vi "mul_add_24_dc_ht_reg.vi"(4 "cep":bool, 8 "add":fxp<+/-,24,16> format="%#_10g", 10 "Signal":fxp<+/-,24,16>=32.0, 11 "coeff":fxp<+/-,18,2>=0.5) -> (1 "out":fxp<+/-,24,16>)   [LabVIEW 2018]
uses:
  <vilib>/rvi/FXPMathLib/basic elements/DSP48E/simVIs/niFpgaDsp48eSimulationState.ctl
  <vilib>/rvi/FXPMathLib/basic elements/DSP48E/subVIs/niFpgaDsp48eType.ctl
  <vilib>/rvi/FXPMathLib/basic elements/DSP48E/subVIs/niFpgaDsp48eAlumodeOpmodeCarryinselState.ctl
  <vilib>/rvi/FXPMathLib/basic elements/DSP48E/subVIs/niFpgaDsp48eUseMultiplierState.ctl
  <vilib>/rvi/FXPMathLib/basic elements/DSP48E/subVIs/niFpgaDsp48eLogicUnitModeState.ctl
  <vilib>/rvi/FXPMathLib/basic elements/DSP48E/subVIs/niFpgaDsp48eSelectPatternState.ctl
  <vilib>/rvi/FXPMathLib/basic elements/DSP48E/subVIs/niFpgaDsp48eSelectMaskState.ctl
  <vilib>/rvi/FXPMathLib/basic elements/DSP48E/subVIs/niFpgaDsp48eAutoresetState.ctl
  <vilib>/rvi/FXPMathLib/basic elements/DSP48E/simVIs/niFpgaDsp48eResets.ctl
  <vilib>/rvi/FXPMathLib/basic elements/DSP48E/simVIs/niFpgaDsp48eRegisters.ctl
  <vilib>/rvi/FXPMathLib/basic elements/DSP48E/simVIs/niFpgaDsp48eCheckMode.vi
  <vilib>/rvi/FXPMathLib/basic elements/DSP48E/simVIs/niFpgaDsp48eReportInvalidMode.vi
  <vilib>/rvi/FXPMathLib/basic elements/DSP48E/simVIs/niFpgaDsp48eSimBundleEnables.vi
  <vilib>/rvi/FXPMathLib/basic elements/DSP48E/simVIs/niFpgaDsp48eSimMultiplier.vi
  <vilib>/rvi/FXPMathLib/basic elements/DSP48E/simVIs/niFpgaDsp48eSimArithmetic.vi
  <vilib>/rvi/FXPMathLib/basic elements/DSP48E/simVIs/niFpgaDsp48eSimPatternDetect.vi
  <vilib>/rvi/FXPMathLib/basic elements/DSP48E/simVIs/niFpgaDsp48eSimP.vi
  <vilib>/rvi/FXPMathLib/basic elements/DSP48E/simVIs/niFpgaDsp48eSimUpdateState.vi
  <vilib>/rvi/FXPMathLib/basic elements/DSP48E/XNode/niFpgaDsp48e.xnode
panel:
  out "appended array 2":bool[](array[boolean])
  out "appended array":bool[](array[boolean])
  out "number":fxp<+/-,30,16>
  in  "Signal 2":fxp<+/-,24,16>=32.0
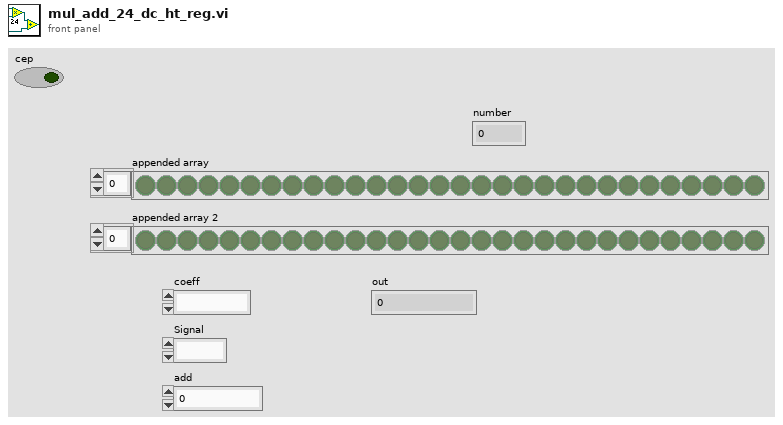
[diagram p1: front panel]
types:
  T1 = cluster{"Boolean array[0]":bool, "Boolean array[1]":bool, "Boolean array[2]":bool, "Boolean array[3]":bool, "Boolean array[4]":bool, "Boolean array[5]":bool, "Boolean array[6]":bool, "Boolean array[7]":bool, "Boolean array[8]":bool, "Boolean array[9]":bool, "Boolean array[10]":bool, "Boolean array[11]":bool, "Boolean array[12]":bool, "Boolean array[13]":bool, "Boolean array[14]":bool, "Boolean array[15]":bool, "Boolean array[16]":bool, "Boolean array[17]":bool, "Boolean array[18]":bool, "Boolean array[19]":bool, "Boolean array[20]":bool, "Boolean array[21]":bool, "Boolean array[22]":bool, "Boolean array[23]":bool}
  T2 = cluster{"Boolean array[0]":bool, "Boolean array[1]":bool, "Boolean array[2]":bool, "Boolean array[3]":bool, "Boolean array[4]":bool, "Boolean array[5]":bool, "Boolean array[6]":bool, "Boolean array[7]":bool, "Boolean array[8]":bool, "Boolean array[9]":bool, "Boolean array[10]":bool, "Boolean array[11]":bool, "Boolean array[12]":bool, "Boolean array[13]":bool, "Boolean array[14]":bool, "Boolean array[15]":bool, "Boolean array[16]":bool, "Boolean array[17]":bool}
  T3 = cluster{"Boolean array[0]":bool, "Boolean array[1]":bool, "Boolean array[2]":bool, "Boolean array[3]":bool, "Boolean array[4]":bool, "Boolean array[5]":bool, "Boolean array[6]":bool, "Boolean array[7]":bool, "Boolean array[8]":bool, "Boolean array[9]":bool, "Boolean array[10]":bool, "Boolean array[11]":bool, "Boolean array[12]":bool, "Boolean array[13]":bool, "Boolean array[14]":bool, "Boolean array[15]":bool, "Boolean array[16]":bool, "Boolean array[17]":bool, "Boolean array[18]":bool, "Boolean array[19]":bool, "Boolean array[20]":bool, "Boolean array[21]":bool, "Boolean array[22]":bool, "Boolean array[23]":bool, "Boolean array[24]":bool, "Boolean array[25]":bool, "Boolean array[26]":bool, "Boolean array[27]":bool, "Boolean array[28]":bool, "Boolean array[29]":bool, "Boolean array[30]":bool, "Boolean array[31]":bool, "Boolean array[32]":bool, "Boolean array[33]":bool, "Boolean array[34]":bool, "Boolean array[35]":bool, "Boolean array[36]":bool, "Boolean array[37]":bool, "Boolean array[38]":bool, "Boolean array[39]":bool, "Boolean array[40]":bool, "Boolean array[41]":bool, "Boolean array[42]":bool, "Boolean array[43]":bool, "Boolean array[44]":bool, "Boolean array[45]":bool, "Boolean array[46]":bool, "Boolean array[47]":bool}
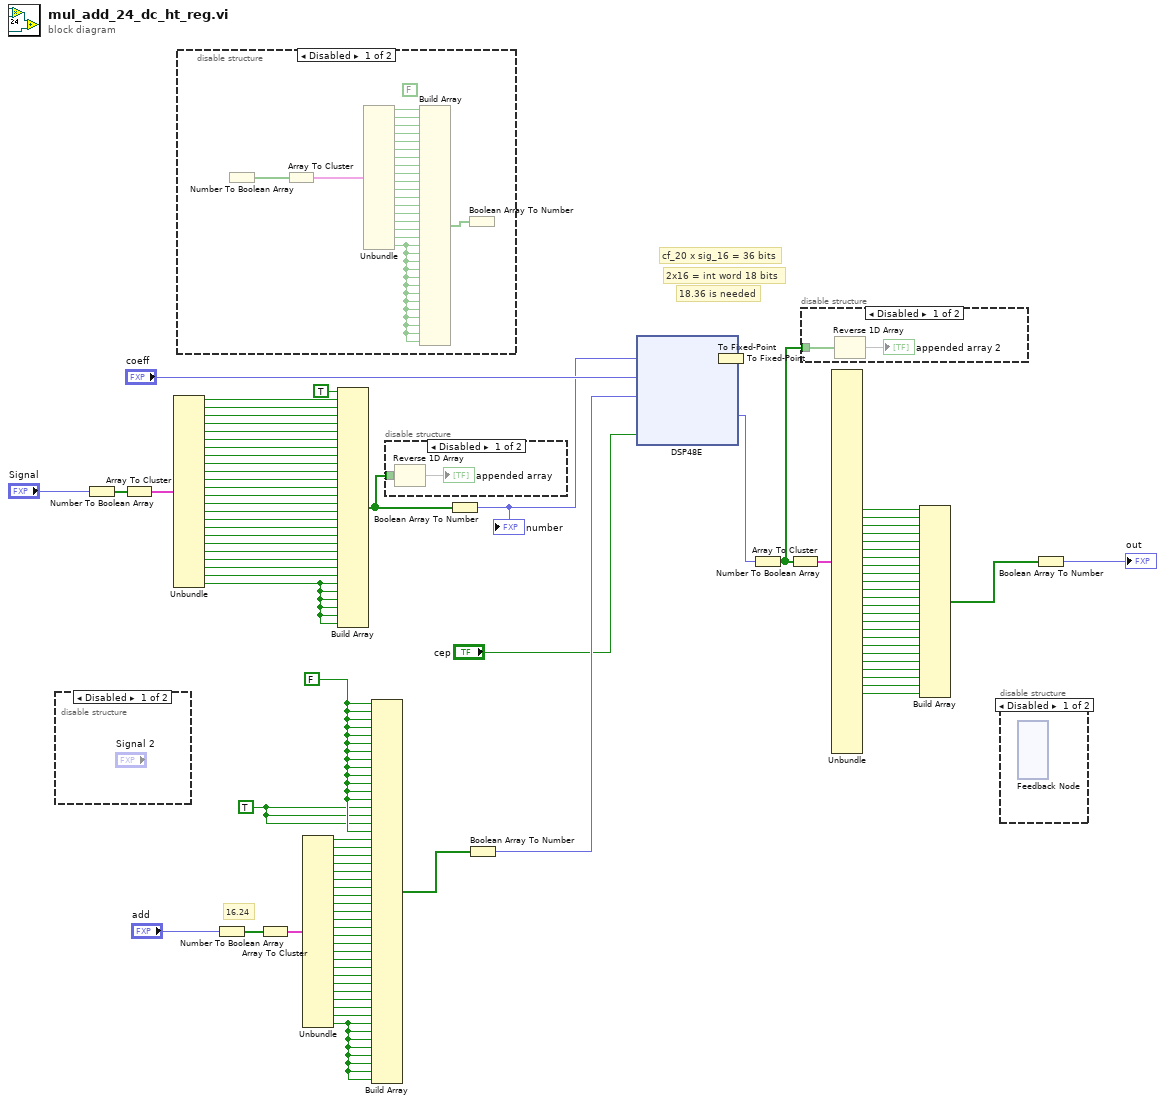
[diagram p0: block diagram]
diagram:
  w3 = TRUE ("element")
  w6 = FALSE ("Boolean array[0]")
  # "16.24"
  # "18.36 is needed"
  # "2x16 = int word 18 bits"
  # "cf_20 x sig_16 = 36 bits"
  n1 = disable-structure shown="Disabled" {
    frame Disabled {
    }
    frame Enabled {
    }
  }
  n2 = Number To Boolean Array(number="Signal") -> (Boolean array=w30:bool[])
  n3 = Array To Cluster(array=w30) -> (cluster=w94:T1)
  n4 = Unbundle(w94) -> ("Boolean array[0]"=w28:bool, "Boolean array[1]"=w27:bool, "Boolean array[2]"=w26:bool, "Boolean array[3]"=w25:bool, "Boolean array[4]"=w24:bool, "Boolean array[5]"=w23:bool, "Boolean array[6]"=w93:bool, "Boolean array[7]"=w92:bool, "Boolean array[8]"=w91:bool, "Boolean array[9]"=w90:bool, "Boolean array[10]"=w89:bool, "Boolean array[11]"=w88:bool, "Boolean array[12]"=w87:bool, "Boolean array[13]"=w86:bool, "Boolean array[14]"=w85:bool, "Boolean array[15]"=w84:bool, "Boolean array[16]"=w47:bool, "Boolean array[17]"=w46:bool, "Boolean array[18]"=w41:bool, "Boolean array[19]"=w42:bool, "Boolean array[20]"=w43:bool, "Boolean array[21]"=w44:bool, "Boolean array[22]"=w45:bool, "Boolean array[23]"=w16:bool)
  n5 = disable-structure shown="Disabled" {
    frame Disabled {
      (unwired) FALSE ("Boolean array[0]")
      n6 = Number To Boolean Array() -> (Boolean array=w96:bool[])  [unwired: 1 in]
      n7 = Array To Cluster(array=w96) -> (cluster=w98:T2)
      n8 = Unbundle(w98) -> ("Boolean array[0]"=w99:bool, "Boolean array[1]"=w115:bool, "Boolean array[2]"=w100:bool, "Boolean array[3]"=w101:bool, "Boolean array[4]"=w102:bool, "Boolean array[5]"=w103:bool, "Boolean array[6]"=w104:bool, "Boolean array[7]"=w105:bool, "Boolean array[8]"=w106:bool, "Boolean array[9]"=w107:bool, "Boolean array[10]"=w108:bool, "Boolean array[11]"=w109:bool, "Boolean array[12]"=w110:bool, "Boolean array[13]"=w111:bool, "Boolean array[14]"=w112:bool, "Boolean array[15]"=w113:bool, "Boolean array[16]"=w114:bool, "Boolean array[17]"=w95:bool)
      n9 = Build Array(w99, w115, w100, w101, w102, w103, w104, w105, w106, w107, w108, w109, w110, w111, w112, w113, w114, w95, w95, w95, w95, w95, w95, w95, w95, w95, w95, w95, w95, w95) -> (w97:bool[])
      n10 = Boolean Array To Number(Boolean array=w97) -> ()  [unwired: 1 out]
    }
    frame Enabled {
    }
  }
  n11 = Number To Boolean Array(number="add") -> (Boolean array=w83:bool[])
  n12 = Array To Cluster(array=w83) -> (cluster=w82:T1)
  n13 = Unbundle(w82) -> ("Boolean array[0]"=w59:bool, "Boolean array[1]"=w60:bool, "Boolean array[2]"=w61:bool, "Boolean array[3]"=w62:bool, "Boolean array[4]"=w63:bool, "Boolean array[5]"=w64:bool, "Boolean array[6]"=w65:bool, "Boolean array[7]"=w66:bool, "Boolean array[8]"=w67:bool, "Boolean array[9]"=w68:bool, "Boolean array[10]"=w69:bool, "Boolean array[11]"=w70:bool, "Boolean array[12]"=w71:bool, "Boolean array[13]"=w72:bool, "Boolean array[14]"=w73:bool, "Boolean array[15]"=w74:bool, "Boolean array[16]"=w75:bool, "Boolean array[17]"=w76:bool, "Boolean array[18]"=w77:bool, "Boolean array[19]"=w78:bool, "Boolean array[20]"=w79:bool, "Boolean array[21]"=w80:bool, "Boolean array[22]"=w81:bool, "Boolean array[23]"=w7:bool)
  n14 = Build Array(TRUE ("element"), w28, w27, w26, w25, w24, w23, w93, w92, w91, w90, w89, w88, w87, w86, w85, w84, w47, w46, w41, w42, w43, w44, w45, w16, w16, w16, w16, w16, w16) -> (w18:bool[])
  n15 = Build Array(w6, w6, w6, w6, w6, w6, w6, w6, w6, w6, w6, w6, w6, w3, w3, w3, w6, w59, w60, w61, w62, w63, w64, w65, w66, w67, w68, w69, w70, w71, w72, w73, w74, w75, w76, w77, w78, w79, w80, w81, w7, w7, w7, w7, w7, w7, w7, w7) -> (w33:bool[])
  n16 = disable-structure shown="Disabled" {
    disable-tunnel: w18 -> [w117 _]
    frame Disabled {
      n17 = Reverse 1D Array(array=w117) -> (reversed array=→"appended array":bool[])
    }
    frame Enabled {
    }
  }
  n18 = Boolean Array To Number(Boolean array=w18) -> (number=w22:fxp<+/-,30,16>)
  "number" <- w22
  n19 = Boolean Array To Number(Boolean array=w33) -> (number=w8:fxp<+/-,48,18>)
  n20 = To Fixed-Point(number=w22) -> (fixed-point=w1:fxp<+/-,30,16>)  [unwired: 1 in]
  n21 = To Fixed-Point(number=w1) -> (fixed-point=w2:fxp<+/-,25,11>)  [unwired: 1 in]
  n22 = xnode ("DSP48E")("a"=w2, "b"="coeff", "c"=w8, "cep"="cep") -> ("p"=w40:fxp<+/-,48,48>)
  n23 = Number To Boolean Array(number=w40) -> (Boolean array=w17:bool[])
  n24 = Array To Cluster(array=w17) -> (cluster=w58:T3)
  n25 = disable-structure shown="Disabled" {
    disable-tunnel: w17 -> [w118 _]
    frame Disabled {
      n26 = Reverse 1D Array(array=w118) -> (reversed array=→"appended array 2":bool[])
    }
    frame Enabled {
    }
  }
  n27 = Unbundle(w58) -> ("Boolean array[17]"=w15:bool, "Boolean array[18]"=w14:bool, "Boolean array[19]"=w13:bool, "Boolean array[20]"=w12:bool, "Boolean array[21]"=w11:bool, "Boolean array[22]"=w10:bool, "Boolean array[23]"=w9:bool, "Boolean array[24]"=w51:bool, "Boolean array[25]"=w52:bool, "Boolean array[26]"=w53:bool, "Boolean array[27]"=w54:bool, "Boolean array[28]"=w55:bool, "Boolean array[29]"=w56:bool, "Boolean array[30]"=w57:bool, "Boolean array[31]"=w48:bool, "Boolean array[32]"=w49:bool, "Boolean array[33]"=w50:bool, "Boolean array[34]"=w39:bool, "Boolean array[35]"=w38:bool, "Boolean array[36]"=w32:bool, "Boolean array[37]"=w31:bool, "Boolean array[38]"=w20:bool, "Boolean array[39]"=w21:bool, "Boolean array[40]"=w19:bool)  [unwired: 24 out]
  n28 = Build Array(w15, w14, w13, w12, w11, w10, w9, w51, w52, w53, w54, w55, w56, w57, w48, w49, w50, w39, w38, w32, w31, w20, w21, w19) -> (w37:bool[])
  n29 = disable-structure shown="Disabled" {
    frame Disabled {
      n30 = feedback #1() -> ()  [unwired: 2 in]
      n31 = feedback-in #1() -> ()  [unwired: 1 in, 1 out]
    }
    frame Enabled {
    }
  }
  n32 = Boolean Array To Number(Boolean array=w37) -> (number=→"out":fxp<+/-,24,16>)
